vi "CFG Determine Numeric Type.vi"(0 "Format String":string) -> (4 "Float":bool)   [LabVIEW 2012]
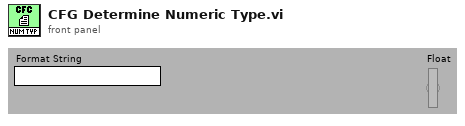
[diagram p1: front panel]
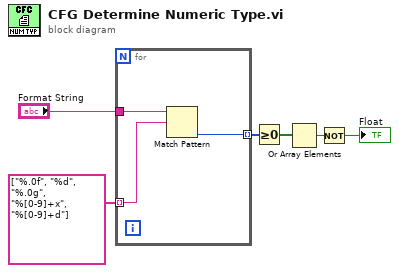
[diagram p0: block diagram]
diagram:
  n1 = for {
    tunnel: "Format String" -> [w9]
    tunnel: string[] ["%.0f", "%d", "%.0g", "%[0-9]+x", "%[0-9]+d"] -> [w8] mode=indexing
    tunnel: [w7] -> w4 mode=indexing
    n2 = Match Pattern(string=w9, regular expression=w8) -> (offset past match=w7:i32)  [unwired: 4 out]
  }
  n3 = Greater Or Equal To 0?(x=w4) -> (x >= 0?=w3:bool[])
  n4 = Or Array Elements(Boolean array=w3) -> (logical OR=w2:bool)
  n5 = Not(x=w2) -> (.not. x?=→"Float":bool)
